vi "Build.vi"(8 "error in (no error)":errorcluster, 11 "Column Factory in":refnum<class "Column Factory.lvclass">) -> (0 "error out":errorcluster, 2 "Column":refnum<class "Column Interface.lvclass">, 3 "Column Factory out":refnum<class "Column Factory.lvclass">)   [LabVIEW 2020, in "Column Interfaces.lvlib" / "Column Factory.lvclass"]
uses:
  Column Factory.lvclass
  Column Interface/Column Interface Class/Column Interface.lvclass
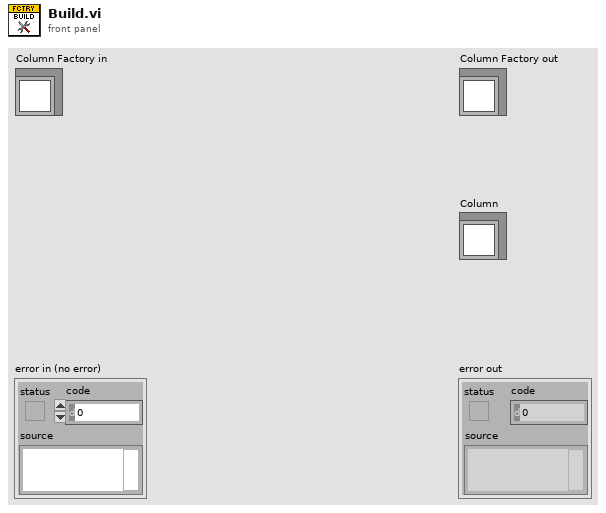
[diagram p1: front panel]
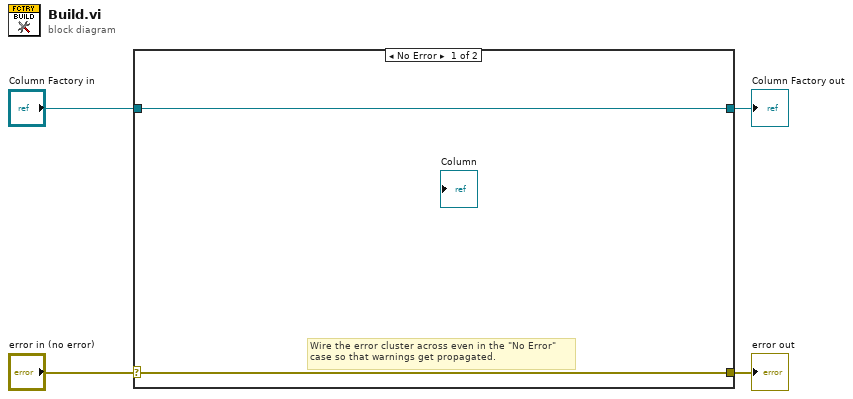
[diagram p0: block diagram]
diagram:
  n1 = case shown="No Error" "error in (no error)" {
    selector: "error in (no error)" -> [w5 w8]
    tunnel: [w5 w8] -> w3
    tunnel: [w6 w7] -> w1
    tunnel: "Column Factory in" -> [w6 w7]
    frame No Error {
      # "Wire the error cluster across even in the \"No Error\"\ncase so that warnings get propagated."
    }
    frame Error {
    }
  }
  "error out" <- w3
  "Column Factory out" <- w1
